vi "FL_DEC_split_2_and_prefilter.vi"(0 "DEC input cluster":T3, 1 "SG filter coefficients":dbl[](array[numeric])) -> (3 "Times":T2, 4 "TTLs":cluster{"TTL in 1":i16, "TTL in 2":i16}, 5 "Magnets coords":cluster{"X1":dbl, "Y1":dbl, "X2":dbl, "Y2":dbl}, 6 "Magnets coords raw":T1)   [LabVIEW 2018, in "Tracker.lvlib"]
uses:
  Tracker.lvlib
  Controls/CTL_Decoded_data_frame.ctl
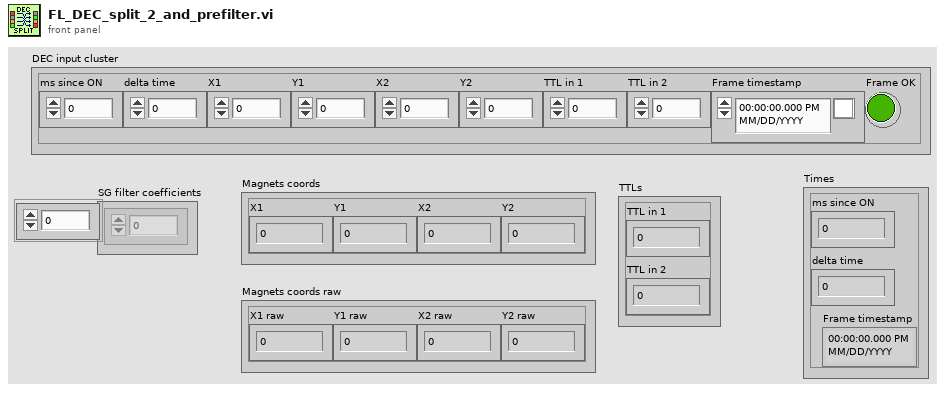
[diagram p1: front panel]
types:
  T1 = cluster{"X1 raw":dbl, "Y1 raw":dbl, "X2 raw":dbl, "Y2 raw":dbl}
  T2 = cluster{"ms since ON":u32, "delta time":u32, "Frame timestamp":timestamp}
  T3 = typedef "Tracker.lvlib/CTL_Decoded_data_frame.ctl" = cluster{"ms since ON":u32, "delta time":u32, "X1":sgl, "Y1":sgl, "X2":sgl, "Y2":sgl, "TTL in 1":i16, "TTL in 2":i16, "Frame timestamp":timestamp, "Frame OK":bool}
  T4 = cluster{"Filtered sample":dbl, "Filtered sample":dbl, "Filtered sample":dbl, "Filtered sample":dbl}
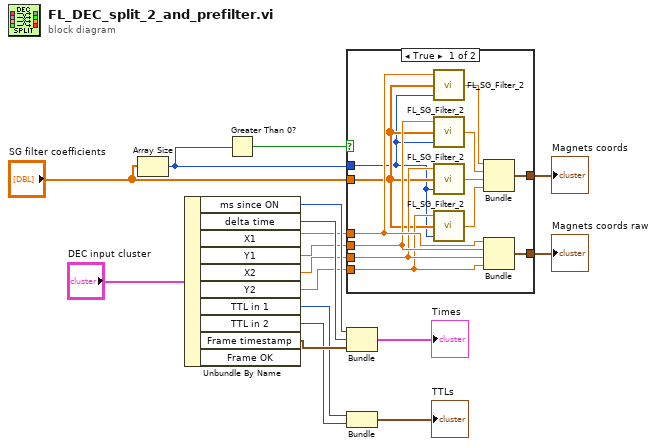
[diagram p0: block diagram]
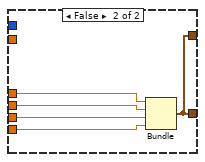
[diagram p2: hidden frame]
diagram:
  n1 = Array Size(array="SG filter coefficients") -> (size(s)=w1:i32)
  n2 = Unbundle By Name("DEC input cluster") -> ("ms since ON"=w16:u32, "delta time"=w15:u32, "X1"=w11:sgl, "Y1"=w10:sgl, "X2"=w9:sgl, "Y2"=w8:sgl, "TTL in 1"=w7:i16, "TTL in 2"=w6:i16, "Frame timestamp"=w14:timestamp)  [unwired: 1 out]
  n3 = Greater Than 0?(x=w1) -> (x > 0?=w2:bool)
  n4 = case shown="True" w2 {
    tunnel: [w25 w30] -> w12
    tunnel: w11 -> [w24 w34]
    tunnel: w10 -> [w23 w33]
    tunnel: w9 -> [w22 w32]
    tunnel: w8 -> [w21 w31]
    tunnel: "SG filter coefficients" -> [w20 _]
    tunnel: [w19 w30] -> w3
    tunnel: w1 -> [w18 _]
    frame True {
      n5 = call "FL_SG_Filter_2.vi"("N samples"=w18, "SG coefficients"=w20, "Input sample"=w24) -> ("Filtered sample"=w29:dbl)
      n6 = call "FL_SG_Filter_2.vi"("N samples"=w18, "SG coefficients"=w20, "Input sample"=w23) -> ("Filtered sample"=w28:dbl)
      n7 = call "FL_SG_Filter_2.vi"("N samples"=w18, "SG coefficients"=w20, "Input sample"=w22) -> ("Filtered sample"=w27:dbl)
      n8 = call "FL_SG_Filter_2.vi"("N samples"=w18, "SG coefficients"=w20, "Input sample"=w21) -> ("Filtered sample"=w26:dbl)
      n9 = Bundle("Filtered sample"=w29, "Filtered sample"=w28, "Filtered sample"=w27, "Filtered sample"=w26) -> (w25:T4)  [unwired: 1 in]
      n10 = Bundle("X1"=w24, "Y1"=w23, "X2"=w22, "Y2"=w21) -> (w19:cluster{"X1":sgl, "Y1":sgl, "X2":sgl, "Y2":sgl})  [unwired: 1 in]
    }
    frame False {
      n11 = Bundle("X1"=w34, "Y1"=w33, "X2"=w32, "Y2"=w31) -> (w30:cluster{"X1":sgl, "Y1":sgl, "X2":sgl, "Y2":sgl})  [unwired: 1 in]
    }
  }
  "Magnets coords" <- w12
  "Magnets coords raw" <- w3
  n12 = Bundle("ms since ON"=w16, "delta time"=w15, "Frame timestamp"=w14) -> (→"Times":T2)  [unwired: 1 in]
  n13 = Bundle("TTL in 1"=w7, "TTL in 2"=w6) -> (→"TTLs":cluster{"TTL in 1":i16, "TTL in 2":i16})  [unwired: 1 in]
